vi "Configure Serial Bus (SPI - Trigger).vi"(0 "VISA resource name":refnum<visa-resource-name>, 1 "MISO Data Pattern (XXXXXXXX)":string="XXXXXXXX", 2 "MOSI Data Pattern (XXXXXXXX)":string="XXXXXXXX", 5 "Serial Bus Name (1: Serial Bus 1)":i32(ring)=1 items=["Serial Bus 1"=1, "Serial Bus 2"=2], 7 "MISO Data Length (8 bits)":i32=8, 9 "Trigger Type (0: MOSI)":i32(ring) items=["MOSI", "MISO"], 11 "error in (no error)":errorcluster, 12 "MOSI Data Length (8 bits)":i32=8) -> (4 "VISA resource name out":refnum<visa-resource-name>, 15 "error out":errorcluster)   [LabVIEW 2016, in "Agilent 2000 3000 X-Series.lvlib"]
doc: "Configures the trigger settings of SPI bus."
uses:
  Agilent 2000 3000 X-Series.lvlib
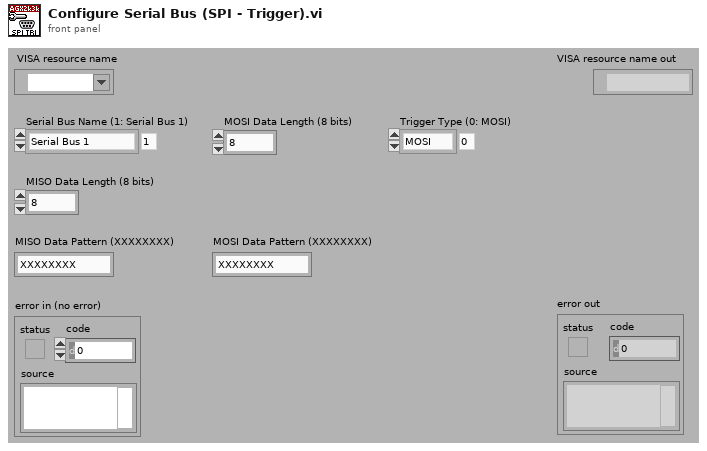
[diagram p1: front panel]
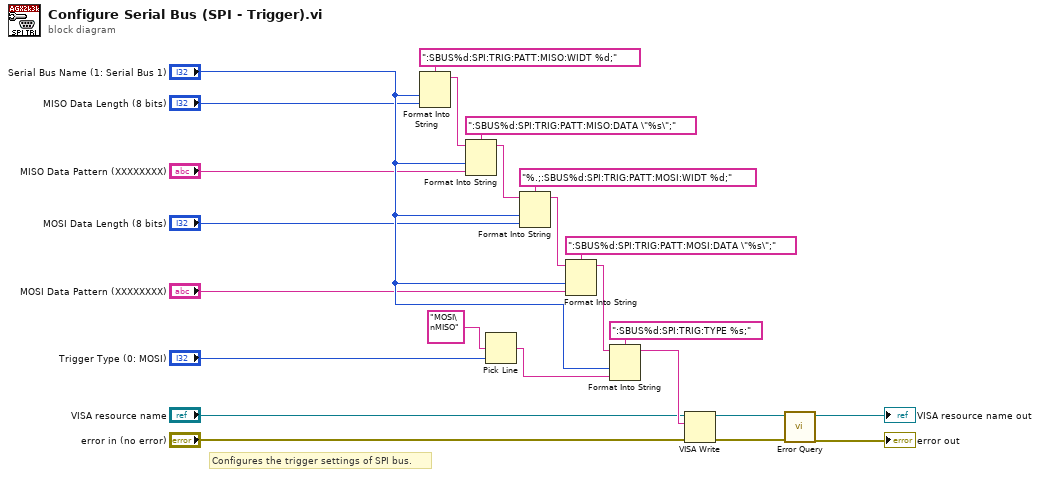
[diagram p0: block diagram]
diagram:
  # "Configures the trigger settings of SPI bus."
  n1 = Format Into String(format string=":SBUS%d:SPI:TRIG:PATT:MISO:WIDT %d;", "Serial Bus Name (1: Serial Bus 1)", "MISO Data Length (8 bits)") -> (resulting string=w4:string)  [unwired: 2 in, 1 out]
  n2 = Format Into String(format string=":SBUS%d:SPI:TRIG:PATT:MISO:DATA \"%s\";", initial string=w4, "Serial Bus Name (1: Serial Bus 1)", "MISO Data Pattern (XXXXXXXX)") -> (resulting string=w3:string)  [unwired: 1 in, 1 out]
  n3 = Pick Line(multi-line string="MOSI\nMISO", line index="Trigger Type (0: MOSI)") -> (output string=w12:string)  [unwired: 1 out]
  n4 = Format Into String(format string="%.;:SBUS%d:SPI:TRIG:PATT:MOSI:WIDT %d;", initial string=w3, "Serial Bus Name (1: Serial Bus 1)", "MOSI Data Length (8 bits)") -> (resulting string=w2:string)  [unwired: 1 in, 1 out]
  n5 = Format Into String(format string=":SBUS%d:SPI:TRIG:PATT:MOSI:DATA \"%s\";", initial string=w2, "Serial Bus Name (1: Serial Bus 1)", "MOSI Data Pattern (XXXXXXXX)") -> (resulting string=w1:string)  [unwired: 1 in, 1 out]
  n6 = Format Into String(format string=":SBUS%d:SPI:TRIG:TYPE %s;", initial string=w1, "Serial Bus Name (1: Serial Bus 1)", w12) -> (resulting string=w11:string)  [unwired: 1 in, 1 out]
  n7 = VISA Write(VISA resource name="VISA resource name", write buffer=w11, error in (no error)="error in (no error)") -> (VISA resource name out=w8:refnum<visa-resource-name>, error out=w7:errorcluster)  [unwired: 1 out]
  n8 = call "Error Query.vi"("error in (no error)"=w7, "VISA resource name"=w8) -> ("error out"=→"error out":errorcluster, "VISA resource name out"=→"VISA resource name out":refnum<visa-resource-name>)  [unwired: 8 out]
